vi "GetHelp.vi"(11 "ExecuteBuildSpec in":refnum<class "ExecuteBuildSpec.lvclass">) -> (2 "Help":string, 3 "ExecuteBuildSpec out":refnum<class "ExecuteBuildSpec.lvclass">)   [LabVIEW 2014, in "ExecuteBuildSpec.lvclass"]
uses:
  ExecuteBuildSpec.lvclass
panel:
  in  "Help":string="LabVIEWCLI -OperationName ExecuteBuildSpec -ProjectPath <path of LabVIEW project>  [-BuildSpecName <name of the build specification>]  [-TargetName <name of the target>]\n\n -ProjectPath : Specifies the full path to the LabVIEW project (.lvproj) file that contains the build specification. \n -BuildSpecName : Specifies the name of the build specification. Enter the name that appears under Build Specifications in the Project Explorer window to specify which build specification builds. If you do not specify a build specification, the LabVIEWCLI builds all build specifications under the specified target. \n -TargetName : Specifies the target that contains the build specification. The target is \"My Computer\" by default. \n"
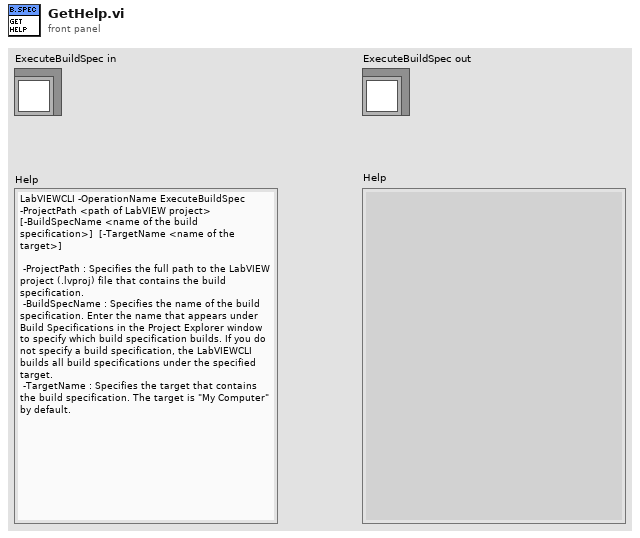
[diagram p1: front panel]
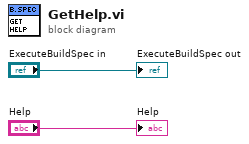
[diagram p0: block diagram]
diagram:
  "ExecuteBuildSpec out" <- "ExecuteBuildSpec in"
  "Help" <- "Help"
